vi "Settings.vi"() -> ()   [LabVIEW 2021, in "Seq Edit Quick Drop.lvlib"]
uses:
  Seq Edit Quick Drop.lvlib
panel:
  in  "Default Shortcut Modifiers":T1
  in  "Main Shortcut":T2={"Key"="SPACE", "Modifiers"={"SHIFT"=TRUE, "CONTROL"=FALSE, "ALT"=FALSE}}
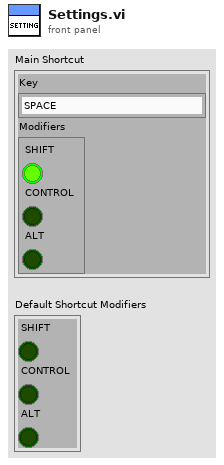
[diagram p1: front panel]
types:
  T1 = cluster{"SHIFT":bool, "CONTROL":bool, "ALT":bool}
  T2 = cluster{"Key":string, "Modifiers":cluster{"SHIFT":bool, "CONTROL":bool, "ALT":bool}}
diagram:
